vi "Sequence Editor Main.vi"() -> ()   [LabVIEW 2015, in "Configuration Tool.lvlib"]
doc: "This is the main VI for the configuration editor.Copyright 2017 National Instruments Corporation\n\nLicensed under the Apache License, Version 2.0 (the \"License\"); you may not use this file except in compliance with the License. You may obtain a copy of the License at http://www.apache.org/licenses/LICENSE-2.0\nUnless required by applicable law or agreed to in writing, software distributed under the License is distributed on an \"AS IS\" BASIS, WITHOUT WARRANTIES OR CONDITIONS OF ANY KIND, either express or implied. See the License for the specific language governing permissions and limitations under the License."
uses:
  Configuration Tool.lvlib
  Controls/StateCluster.ctl
  <vilib>/NI/Configuration Framework/Repository/NISE_CEF_Repository.lvclass
  <vilib>/NI/Configuration Framework/Node/NodeRef.ctl
  <vilib>/NI/Configuration Framework/Node/NISE_CEF_Node.lvclass
  <vilib>/NI/Configuration Framework/Node/StandardEvents.ctl
  <vilib>/NI/Configuration Framework/Node/UserEventRef.ctl
  <vilib>/NI/Configuration Framework/Controls/EventCluster.ctl
  <vilib>/NI/Configuration Framework/Node/NodeChangeEvent.ctl
  <vilib>/NI/Configuration Framework/Node/CacheState.ctl
  <vilib>/NI/Configuration Framework/Node/RefreshUIEvent.ctl
  <vilib>/NI/Configuration Framework/Node/StopEvent.ctl
  <vilib>/NI/Configuration Framework/glyph manager/glyph manager.ctl
  <vilib>/picture/picture.llb/imagedata.ctl
  Controls/StepClassLibrary.ctl
  Prototype/classes/Step/Config/Step Config.lvclass
  Prototype/classes/Step/UI/Step UI.lvclass
  Controls/AddMessage.ctl
  Controls/MoveMessage.ctl
  <vilib>/Utility/error.llb/DialogType.ctl
  Classes/SequenceNode/SequenceNode.lvclass
  Classes/SequenceRepo/SequenceRepo.lvclass
  <vilib>/Utility/sysdir.llb/System Directory Type.ctl
  Classes/StepNode/StepNode.lvclass
  <vilib>/NI/AMC/Read Termination Message.vi
  <vilib>/NI/AMC/Create Single Message.vi
  <vilib>/NI/AMC/Update Message Routing Info.vi
  <vilib>/NI/AMC/Send Message.vi
  <vilib>/NI/AMC/Globals.vi
  <vilib>/NI/AMC/AMC.lvlib
  <vilib>/NI/Configuration Framework/NISE_CEF_TreeControl.lvlib
  <vilib>/NI/Configuration Framework/glyph manager/glyph manager.lvlib
panel:
  in  "View":string(tree)
  in  "Exit":bool
  # "Configurator"
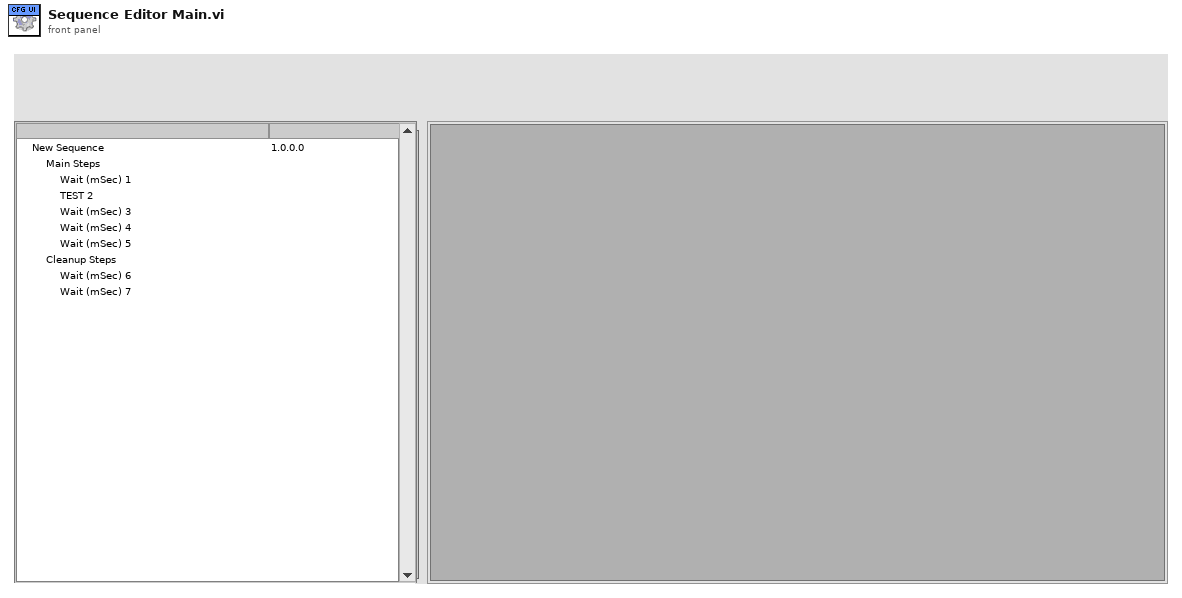
[diagram p1: front panel]
types:
  T1 = typedef "Configuration Tool.lvlib/StateCluster.ctl" = cluster{"repository":refnum<class "NISE_CEF_Repository.lvclass">, "root":T2, "unsaved changes":bool, "current path":path, "standard events":T3, "classes path":path, "glyph manager":T9, "Step Class Library":T11}
  T2 = typedef "NISE_CEF_Node.lvclass/NodeRef.ctl" = refnum<data-value>
  T3 = typedef "NISE_CEF_Node.lvclass/StandardEvents.ctl" = cluster{"user event":T4, "node change":T5, "cache state":T6, "refresh UI":T7, "stop event":T8}
  T4 = typedef "NISE_CEF_Node.lvclass/UserEventRef.ctl" = refnum<user-event>
  T5 = typedef "NISE_CEF_Node.lvclass/NodeChangeEvent.ctl" = refnum<user-event>
  T6 = typedef "NISE_CEF_Node.lvclass/CacheState.ctl" = refnum<user-event>
  T7 = typedef "NISE_CEF_Node.lvclass/RefreshUIEvent.ctl" = refnum<user-event>
  T8 = typedef "NISE_CEF_Node.lvclass/StopEvent.ctl" = refnum<user-event>
  T9 = typedef "glyph manager.lvlib/glyph manager.ctl" = cluster{"search paths":path[], "glyph map":variant, "base glyphs":T10[], "desired overlays":string[]}
  T10 = typedef "imagedata.ctl" = cluster{"image type":i32, "image depth":i32, "image":u8[], "mask":u8[], "colors":u32[], "Rectangle":cluster{"left":i16, "top":i16, "right":i16, "bottom":i16}}
  T11 = typedef "Configuration Tool.lvlib/StepClassLibrary.ctl" = cluster{"Step Types":string[], "Step Config Classes":refnum<class "Step Config.lvclass">[], "Step UI Classes":refnum<class "Step UI.lvclass">[]}
  T12 = typedef "AMC.lvlib/Message Queue.ctl" = refnum<queue>
  T13 = typedef "Configuration Tool.lvlib/AddMessage.ctl" = cluster{"node type":string, "to add to":string}
  T14 = typedef "Configuration Tool.lvlib/MoveMessage.ctl" = cluster{"node ref":T2, "new parent":T2, "Index":i32}
  T15 = typedef "Configuration Tool.lvlib/FilePaths.ctl" = cluster{"glyphs":path, "classes":path}
  T16 = typedef "DialogType.ctl" = u16
  T17 = typedef "System Directory Type.ctl" = i32
  T18 = typedef "NISE_CEF_Node.lvclass/Summary.ctl" = cluster{"ID":string, "parent ID":string, "node type":string, "text":string, "additional text":string, "glyph":string, "depth":i32, "glyph overlay":string}
  T19 = typedef "LVPoint32TypeDef.ctl" = cluster{"Horizontal":i32, "Vertical":i32}
  T20 = cluster{"data name":string, "drag data":variant}[]
  T21 = typedef "NISE_CEF_Node.lvclass/NodeMenuOptions.ctl" = cluster{"removable":bool, "movable":bool, "duplicate":bool}
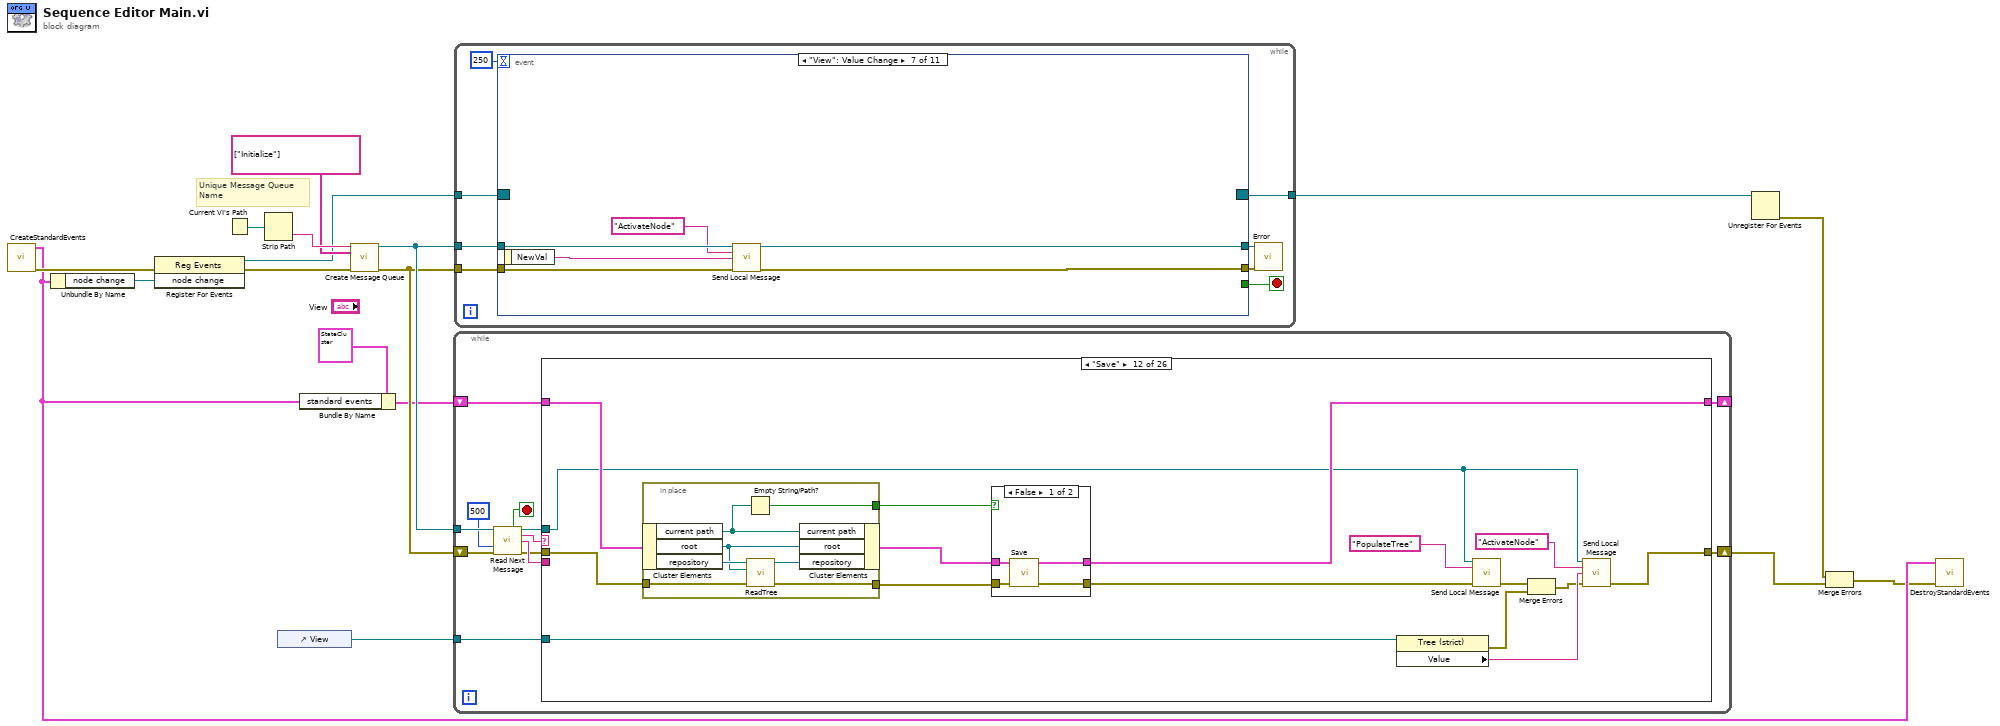
[diagram p0: block diagram]
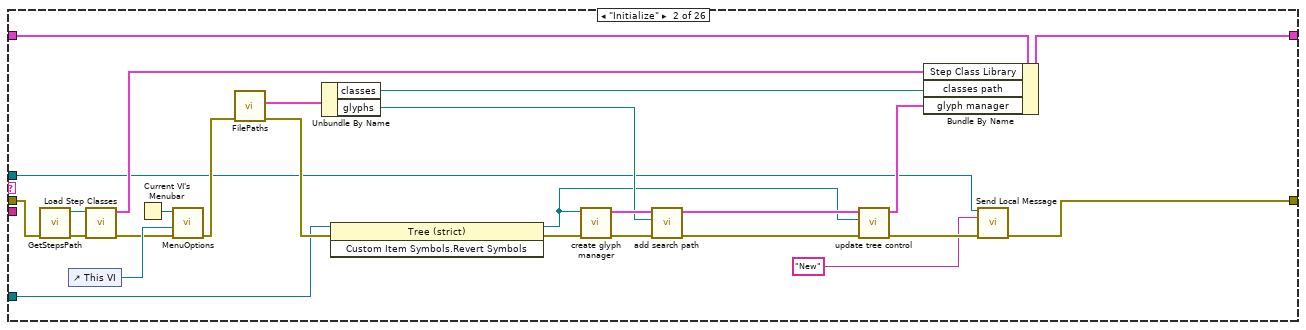
[diagram p3: hidden frame]
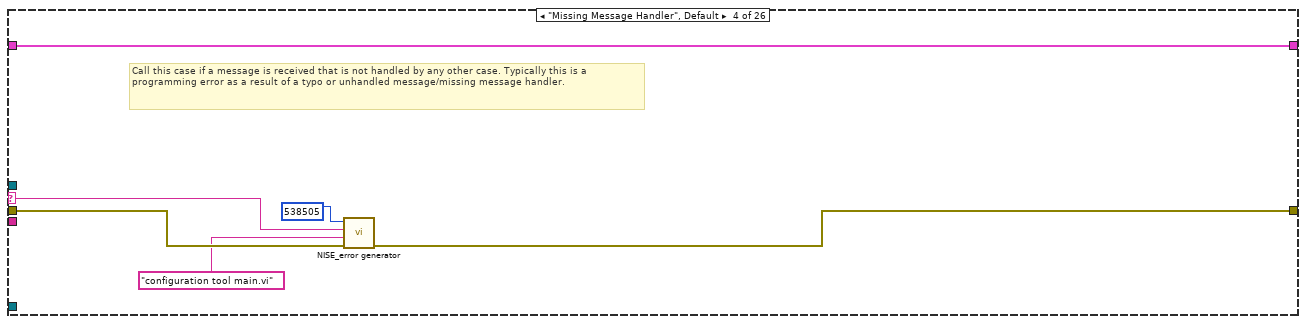
[diagram p5: hidden frame]
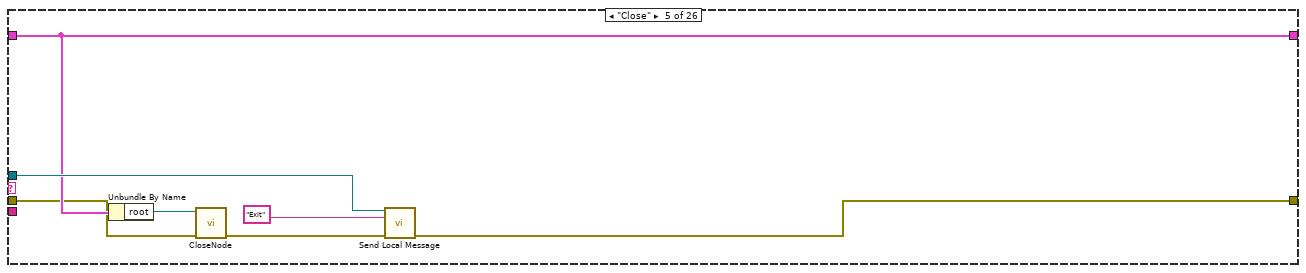
[diagram p6: hidden frame]
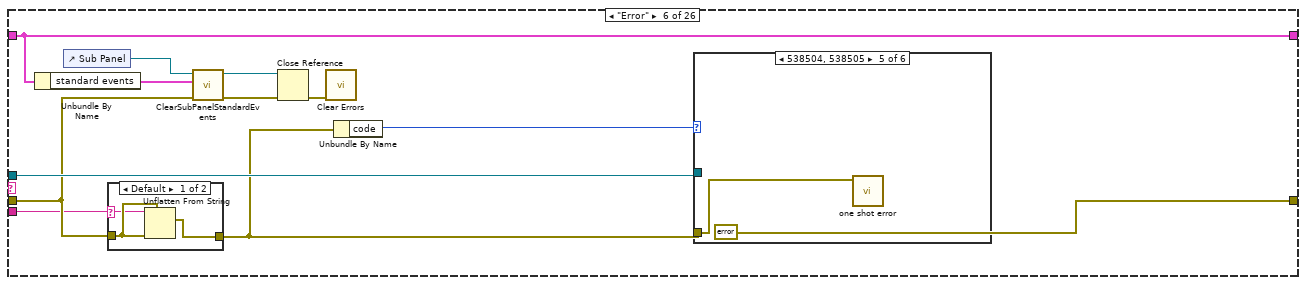
[diagram p7: hidden frame]
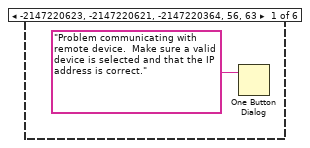
[diagram p9: hidden frame]
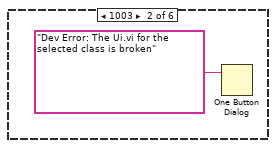
[diagram p10: hidden frame]
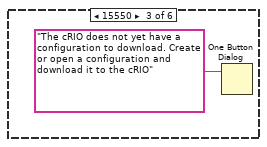
[diagram p11: hidden frame]
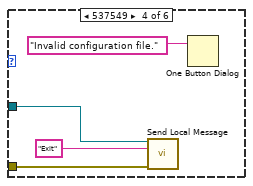
[diagram p12: hidden frame]
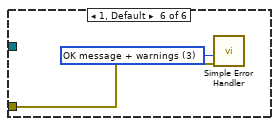
[diagram p13: hidden frame]
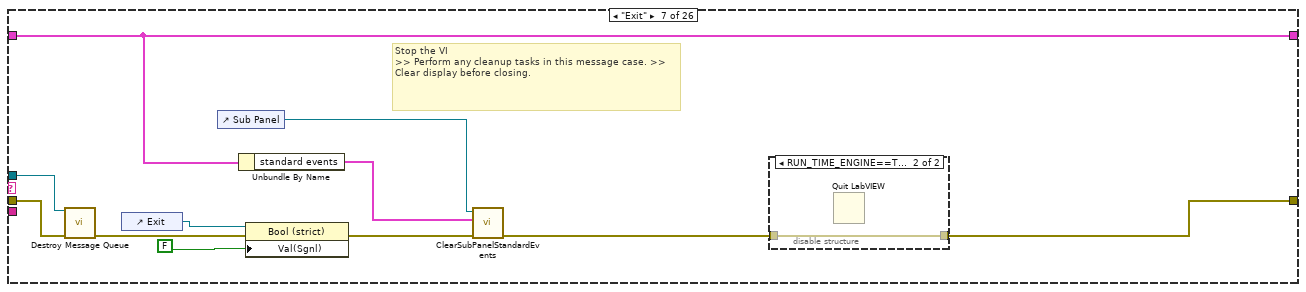
[diagram p14: hidden frame]
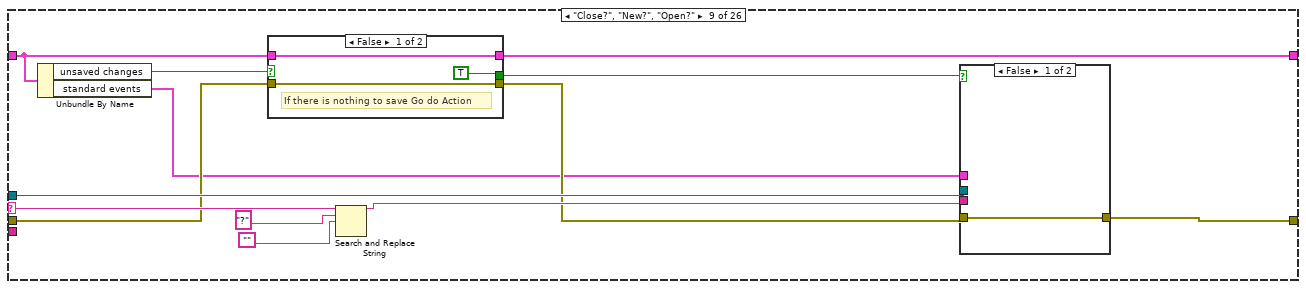
[diagram p17: hidden frame]
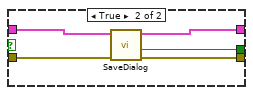
[diagram p18: hidden frame]
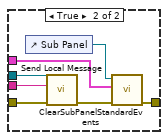
[diagram p19: hidden frame]
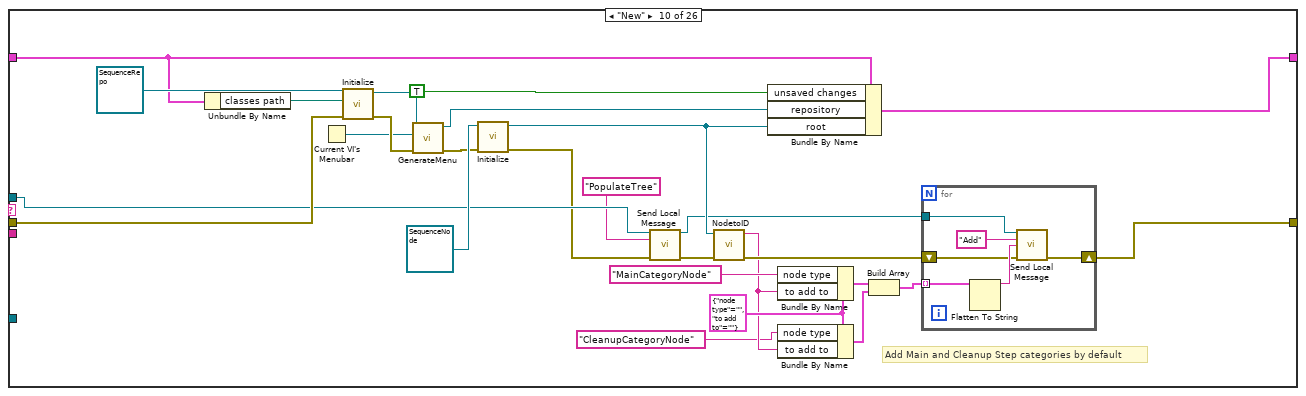
[diagram p20: hidden frame]
diagram:
  # "Unique Message Queue Name"
  n1 = call <vilib>:"CreateStandardEvents.vi"() -> ("error out"=w12:errorcluster, "standard events"=w6:T3)  [unwired: 10 in]
  n2 = Unbundle By Name(w6) -> ("node change"=w11:T5)
  n3 = register-events(error in=w12, w11) -> (reference out=w5:refnum<event-registration>, error out=w10:errorcluster)  [unwired: 1 in]
  n4 = Current VI's Path() -> (path=w16:path)
  n5 = Strip Path(path=w16) -> (name=w17:string)  [unwired: 1 out]
  n6 = control-ref of="View"() -> (w4:refnum<vi>)
  n7 = Bundle By Name(cluster=T1 {"repository"=refnum, "root"=refnum, "unsaved changes"=FALSE, "current path"=path "", "standard events"={"user event"=refnum, "node change"=refnum, "cache state"=refnum, "refresh UI"=refnum, "stop event"=refnum}, "classes path"=path "", "glyph manager"={"search paths"=[], "glyph map"=variant, "base glyphs"=[], "desired overlays"=[]}, "Step Class Library"={"Step Types"=[], "Step Config Classes"=[], "Step UI Classes"=[]}}, "standard events"=w6) -> (w8:T1)
  n8 = call <vilib>:"Create Message Queue.vi"("message queue name"=w17, "initial message names"=string[] ["Initialize"], "error in"=w10) -> ("message queue out"=w14:T12, "error out"=w13:errorcluster)  [unwired: 11 in]
  n9 = while "Message Processor" {
    shift-right: [w25] -> w7
    shift-left: w13 -> [w24]
    tunnel: w14 -> [w23]
    shift-right: [w21] -> _
    shift-left: w8 -> [w20]
    tunnel: w4 -> [w18]
    stop <- w29 stop-if-true
    n10 = call <vilib>:"Read Next Message.vi"("message queue in"=w23, "timeout (1 ms)"=500, "error in"=w24) -> ("exit process?"=w29:bool, "message queue out"=w19:T12, "message name"=w28:string, "message value"=w27:string, "error out"=w26:errorcluster)  [unwired: 5 in, 3 out]
    n11 = case shown="\"Save\"" w28 {
      selector: w28 -> [_ _ _ w61 _ _ _ _ w122 _ _ _ _ _ _ _ _ _ w423 _ _ _ _ _ _ _]
      tunnel: w27 -> [_ _ _ _ _ w74 _ _ _ _ _ _ _ w262 _ w311 w370 w401 w421 w473 w497 _ _ w537 w558 w565]
      tunnel: w26 -> [w31 w35 w59 w64 w67 w77 w109 w113 w115 w163 w182 w229 w254 w269 w282 w303 w365 w400 w426 w475 w496 w518 w527 w536 w556 w566]
      tunnel: [w31 w34 w59 w62 w71 errorcluster {"status"=FALSE, "code"=0, "source"=""} ("error out") w101 w113 w126 w156 w178 w225 w256 w266 w282 w305 w336 w404 w429 w477 w493 w512 w523 w533 w551 w564] -> w25
      tunnel: [w30 w53 w58 w65 w69 w81 w100 w112 w117 w169 w183 w235 w255 w263 w281 w298 w360 w397 w430 w476 w498 w509 w526 w531 w559 w561] -> w21
      tunnel: w20 -> [w30 w54 w58 w65 w69 w81 w100 w112 w118 w165 w184 w231 w253 w264 w281 w301 w363 w398 w430 w468 w498 w521 w526 w531 w559 w567]
      tunnel: w19 -> [_ w33 _ _ w70 w84 w108 _ w125 w154 w180 w223 _ w265 _ _ w335 _ w424 _ _ _ _ w532 w550 w563]
      tunnel: w18 -> [_ w40 _ _ _ _ _ _ _ _ _ w226 _ _ _ w299 w361 w393 w418 w470 w491 w510 _ _ _ _]
      frame "------------Generic Operations------------" {
        # "Dummy case to add a seperation in the Case Structure menu"
      }
      frame "Initialize" {
        n12 = call "GetStepsPath.vi"("error in (no error)"=w35) -> ("error out"=w36:errorcluster, "Steps Folder Path"=w37:path)  [unwired: 9 in]
        n13 = control-ref of="This VI"() -> (w57:refnum<vi>)
        n14 = call "Load Step Classes.vi"("error in (no error)"=w36, "Step Classes Folder Path"=w37) -> ("error out"=w39:errorcluster, "Step Class Library"=w38:T11)  [unwired: 8 in]
        n15 = Current VI's Menubar() -> (w56:refnum<k9>)
        n16 = call "MenuOptions.vi"("error in"=w39, "VI ref"=w57, "menu ref in"=w56) -> ("error out"=w52:errorcluster)  [unwired: 7 in, 1 out]
        n17 = call "FilePaths.vi"("error in"=w52) -> ("error out"=w43:errorcluster, "paths"=w55:T15)  [unwired: 9 in]
        n18 = Unbundle By Name(w55) -> ("classes"=w51:path, "glyphs"=w45:path)
        n19 = invoke class="Tree (strict)" method="Custom Item Symbols.Revert Symbols"(reference=w40, error in=w43) -> (reference out=w41:refnum<vi>, error out=w42:errorcluster)  [unwired: 1 in, 1 out]
        n20 = call <vilib>:"create glyph manager.vi"("error in"=w42, "tree ref (for default symbols)"=w41) -> ("error out"=w50:errorcluster, "glyph manager"=w49:T9)  [unwired: 8 in]
        n21 = call <vilib>:"add search path.vi"("error in"=w50, "search path"=w45, "glyph manager in"=w49) -> ("error out"=w48:errorcluster, "glyph manager out"=w47:T9)  [unwired: 7 in]
        n22 = call <vilib>:"update tree control.vi"("error in"=w48, "tree reference"=w41, "glyph manager in"=w47) -> ("error out"=w46:errorcluster, "glyph manager out"=w44:T9)  [unwired: 7 in]
        n23 = Bundle By Name(cluster=w54, "Step Class Library"=w38, "classes path"=w51, "glyph manager"=w44) -> (w53:T1)
        n24 = call <vilib>:"Send Local Message.vi"("message queue in"=w33, "message name"="New", "error in"=w46) -> ("error out"=w34:errorcluster)  [unwired: 10 in, 2 out]
      }
      frame "", "Idle" {
      }
      frame "Missing Message Handler", Default {
        # "Call this case if a message is received that is not handled by any other case. Typically this is a programming error as a result of a typo or unhandled message/missing message handler."
        n25 = call <vilib>:"NISE_error generator.vi"("error in"=w64, "source"="configuration tool main.vi", "append error message"=w61, "error code (0)"=538505) -> ("error out"=w62:errorcluster)  [unwired: 5 in]
      }
      frame "Close" {
        n26 = Unbundle By Name(w69) -> ("root"=w68:T2)
        n27 = call <vilib>:"CloseNode.vi"("error in"=w67, "node ref"=w68) -> ("error out"=w66:errorcluster)  [unwired: 9 in]
        n28 = call <vilib>:"Send Local Message.vi"("message queue in"=w70, "message name"="Exit", "error in"=w66) -> ("error out"=w71:errorcluster)  [unwired: 10 in, 2 out]
      }
      frame "Error" {
        n29 = Unbundle By Name(w81) -> ("standard events"=w73:T3)
        n30 = control-ref of="Sub Panel"() -> (w80:refnum<vi>)
        n31 = case shown="Default" w74 {
          selector: w74 -> [w86 _]
          tunnel: w77 -> [w87 w88]
          tunnel: [w85 w88] -> w76
          frame Default {
            n32 = Unflatten From String(type=w87, binary string=w86, error in (no error)=w87) -> (value=w85:errorcluster)  [unwired: 2 in, 2 out]
          }
          frame "" {
          }
        }
        n33 = call <vilib>:"ClearSubPanelStandardEvents.vi"("error in"=w77, "standard events"=w73, "sub panel ref in"=w80) -> ("error out"=w79:errorcluster, "sub panel ref out"=w78:refnum<vi>)  [unwired: 7 in]
        n34 = Close Reference(reference=w78, error in (no error)=w79) -> (error out=w75:errorcluster)
        n35 = call <vilib>:"Clear Errors.vi"("error in (no error)"=w75) -> ()  [unwired: 5 in, 2 out]
        n36 = Unbundle By Name(w76) -> ("code"=w82:i32)
        n37 = case shown="538504, 538505" w82 {
          tunnel: w84 -> [_ _ _ w94 _ _]
          tunnel: w76 -> [_ _ _ w93 w96 w98]
          frame -2147220623, -2147220621, -2147220364, 56, 63 {
            n38 = One Button Dialog(message="Problem communicating with remote device.  Make sure a valid device is selected and that the IP address is correct.") -> ()  [unwired: 1 in, 1 out]
          }
          frame 1003 {
            n39 = One Button Dialog(message="Dev Error: The Ui.vi for the selected class is broken") -> ()  [unwired: 1 in, 1 out]
          }
          frame 15550 {
            n40 = One Button Dialog(message="The cRIO does not yet have a configuration to download. Create or open a configuration and download it to the cRIO") -> ()  [unwired: 1 in, 1 out]
          }
          frame 537549 {
            n41 = call <vilib>:"Send Local Message.vi"("message queue in"=w94, "message name"="Exit", "error in"=w93) -> ()  [unwired: 10 in, 3 out]
            n42 = One Button Dialog(message="Invalid configuration file.") -> ()  [unwired: 1 in, 1 out]
          }
          frame 538504, 538505 {
            n43 = call <vilib>:"one shot error.vi"("error in"=w96) -> ()  [unwired: 11 in]
          }
          frame 1, Default {
            w97 = T16 3 items=["no dialog", "OK message", "continue or stop message", "OK message + warnings", "continue/stop + warnings"] ("type of dialog (OK msg:1)")
            n44 = call <vilib>:"Simple Error Handler.vi"("type of dialog (OK msg:1)"=w97, "error in (no error)"=w98) -> ()  [unwired: 8 out]
          }
        }
      }
      frame "Exit" {
        # "Stop the VI                                                                             >> Perform any cleanup tasks in this message case. >> Clear display before closing."
        n45 = call <vilib>:"Destroy Message Queue.vi"("message queue in"=w108, "error in"=w109) -> ("error out"=w105:errorcluster)  [unwired: 11 in, 2 out]
        n46 = control-ref of="Exit"() -> (w107:refnum<vi>)
        n47 = control-ref of="Sub Panel"() -> (w104:refnum<vi>)
        n48 = Unbundle By Name(w100) -> ("standard events"=w99:T3)
        n49 = property class="Bool (strict)"(reference=w107, error in=w105, "Val(Sgnl)"=FALSE ("Exit")) -> (error out=w103:errorcluster)  [unwired: 1 out]
        n50 = call <vilib>:"ClearSubPanelStandardEvents.vi"("error in"=w103, "standard events"=w99, "sub panel ref in"=w104) -> ("error out"=w102:errorcluster)  [unwired: 7 in, 1 out]
        n51 = disable-structure shown="RUN_TIME_ENGINE==True" {
          disable-tunnel: [w110 w111] -> w101
          disable-tunnel: w102 -> [w110 w111]
          frame condition #0 (active) {
          }
          frame condition #1 {
            n52 = Quit LabVIEW() -> ()  [unwired: 1 in]
          }
        }
      }
      frame "------------Menu Operations--------------" {
        # "Dummy case to add a seperation in the Case Structure menu"
      }
      frame "Close?", "New?", "Open?" {
        n53 = Unbundle By Name(w118) -> ("unsaved changes"=w120:bool, "standard events"=w114:T3)
        n54 = case shown="False" w120 {
          tunnel: [TRUE ("SaveFlag") w134] -> w119
          tunnel: w118 -> [w128 w133]
          tunnel: [w128 w132] -> w117
          tunnel: w115 -> [w127 w131]
          tunnel: [w127 w130] -> w116
          frame False {
            # "If there is nothing to save Go do Action"
          }
          frame True {
            n55 = call "SaveDialog.vi"("error in"=w131, "state in"=w133) -> ("error out"=w130:errorcluster, "new"=w134:bool, "state out"=w132:T1)  [unwired: 7 in]
          }
        }
        n56 = Search and Replace String(input string=w122, search string="?", replace string="") -> (result string=w121:string)  [unwired: 5 in, 3 out]
        n57 = case shown="False" w119 {
          tunnel: w116 -> [w135 w142]
          tunnel: [w135 w138] -> w126
          tunnel: w125 -> [_ w141]
          tunnel: w121 -> [_ w140]
          tunnel: w114 -> [_ w136]
          frame False {
          }
          frame True {
            n58 = control-ref of="Sub Panel"() -> (w137:refnum<vi>)
            n59 = call <vilib>:"Send Local Message.vi"("message queue in"=w141, "message name"=w140, "error in"=w142) -> ("error out"=w139:errorcluster)  [unwired: 10 in, 2 out]
            n60 = call <vilib>:"ClearSubPanelStandardEvents.vi"("error in"=w139, "standard events"=w136, "sub panel ref in"=w137) -> ("error out"=w138:errorcluster)  [unwired: 7 in, 1 out]
          }
        }
      }
      frame "New" {
        w146 = T13 {"node type"="", "to add to"=""} ("input cluster")
        # "Add Main and Cleanup Step categories by default"
        n61 = Unbundle By Name(w165) -> ("classes path"=w164:path)
        n62 = Current VI's Menubar() -> (w158:refnum<k9>)
        n63 = call-dynamic "Initialize.vi"("error in"=w163, "path"=w164, "repository in"=refnum<class "SequenceRepo.lvclass"> refnum ("cRIORepo.lvclass")) -> ("error out"=w162:errorcluster, "repository out"=w160:refnum<class "SequenceRepo.lvclass">)  [unwired: 7 in]
        n64 = call-dynamic "GenerateMenu.vi"("error in"=w162, "menu ref in"=w158, "NISE_CEF_Repository in"=w160) -> ("error out"=w161:errorcluster, "NISE_CEF_Repository out"=w159:refnum<class "SequenceRepo.lvclass">)  [unwired: 6 in, 1 out]
        n65 = call-dynamic "Initialize.vi"("error in"=w161, "SequenceNode in"=refnum<class "SequenceNode.lvclass"> refnum ("cRIO.lvclass")) -> ("error out"=w151:errorcluster, "data value reference"=w157:T2)  [unwired: 7 in, 1 out]
        n66 = call <vilib>:"Send Local Message.vi"("message queue in"=w154, "message name"="PopulateTree", "error in"=w151) -> ("message queue out"=w153:T12, "error out"=w150:errorcluster)  [unwired: 10 in, 1 out]
        n67 = call <vilib>:"NodetoID.vi"("error in"=w150, "node ref"=w157) -> ("error out"=w149:errorcluster, "ID"=w144:string)  [unwired: 8 in]
        n68 = Bundle By Name(cluster=w165, "unsaved changes"=TRUE ("SaveFlag"), "repository"=w159, "root"=w157) -> (w169:T1)
        n69 = Bundle By Name(cluster=w146, "node type"="MainCategoryNode", "to add to"=w144) -> (w147:T13)
        n70 = Bundle By Name(cluster=w146, "node type"="CleanupCategoryNode", "to add to"=w144) -> (w145:T13)
        n71 = Build Array(w147, w145) -> (w148:T13[])
        n72 = for {
          tunnel: w148 -> [w173] mode=indexing
          tunnel: w153 -> [w171]
          shift-right: [w175] -> w156
          shift-left: w149 -> [w170]
          n73 = Flatten To String(anything=w173) -> (data string=w172:string)  [unwired: 3 in, 2 out]
          n74 = call <vilib>:"Send Local Message.vi"("message queue in"=w171, "message name"="Add", "message value"=w172, "error in"=w170) -> ("error out"=w175:errorcluster)  [unwired: 9 in, 2 out]
        }
      }
      frame "Open" {
        w177 = T17 0 items=["User Home"=0, "User Desktop"=1, "User Documents"=2, "User Application Data"=3, "User Preferences"=4, "User Temporary"=5, "Public Documents"=6, "Public Application Data"=7, "Public Preferences"=8, "Public Cache"=13, "System Core Libraries"=9, "System Installed Libraries"=10, "Application Files"=11, "Boot Volume Root"=12] ("system directory type")
        n75 = call <vilib>:"Get System Directory.vi"("system directory type"=w177) -> ("system directory"=w176:path)  [unwired: 10 in]
        n76 = in-place {
          in-place-border: w182 -> [w190]
          in-place-border: [w189] -> w179
          in-place-border: w176 -> [w185]
          n77 = in-place-cluster #1(w184) -> ("current path"=w187:path, "repository"=w198:refnum<class "NISE_CEF_Repository.lvclass">, "root"=w194:T2)  [unwired: 1 out]
          n78 = call "FileDialog.vi"("error in"=w190, "start path"=w185) -> ("error out"=w191:errorcluster, "cancelled"=w192:bool, "selected path"=w188:path)  [unwired: 7 in]
          n79 = Compound Arithmetic op=OR(invert w192) -> (w193:bool)
          n80 = case shown="True" w193 {
            tunnel: w198 -> [w199 w211]
            tunnel: [w199 w209] -> w196
            tunnel: [w200 w207] -> w189
            tunnel: [w201 w206] -> w195
            tunnel: w188 -> [_ w204]
            tunnel: w191 -> [w200 w203]
            tunnel: w194 -> [w201 w202]
            frame False {
            }
            frame True {
              n81 = call-dynamic "Open.vi"("error in"=w203, "file path"=w204, "repository in"=w211) -> ("error out"=w208:errorcluster, "invalid?"=w205:bool, "repository out"=w210:refnum<class "NISE_CEF_Repository.lvclass">)  [unwired: 6 in]
              n82 = case shown="False" w205 {
                tunnel: w210 -> [w216 w219]
                tunnel: [w215 w219] -> w209
                tunnel: w208 -> [w214 w218]
                tunnel: [w213 w218] -> w207
                tunnel: [w212 w217] -> w206
                tunnel: w202 -> [_ w217]
                frame False {
                  n83 = call-dynamic "WriteTree.vi"("error in"=w214, "repository in"=w216) -> ("error out"=w213:errorcluster, "root"=w212:T2, "repository out"=w215:refnum<class "NISE_CEF_Repository.lvclass">)  [unwired: 7 in]
                }
                frame True {
                }
              }
            }
          }
          n84 = Select(t=w187, s=w189, f=w188) -> (s? t:f=w186:path)
          n85 = in-place-cluster #1("current path"=w186, "unsaved changes"=FALSE ("SaveFlag"), "repository"=w196, "root"=w195) -> (w183:T1)
        }
        n86 = call <vilib>:"Send Local Message.vi"("message queue in"=w180, "message name"="PopulateTree", "error in"=w179) -> ("error out"=w178:errorcluster)  [unwired: 10 in, 2 out]
      }
      frame "Save" {
        n87 = in-place {
          in-place-border: w229 -> [w239]
          in-place-border: [w238] -> w228
          in-place-border: [w236] -> w227
          n88 = in-place-cluster #2(w231) -> ("current path"=w237:path, "root"=w240:T2, "repository"=w242:refnum<class "NISE_CEF_Repository.lvclass">)
          n89 = Empty String/Path?(string/path=w237) -> (empty?=w236:bool)
          n90 = call-dynamic "ReadTree.vi"("error in"=w239, "root"=w240, "repository in"=w242) -> ("error out"=w238:errorcluster, "repository out"=w241:refnum<class "NISE_CEF_Repository.lvclass">)  [unwired: 7 in]
          n91 = in-place-cluster #2("current path"=w237, "root"=w240, "repository"=w241) -> (w230:T1)
        }
        n92 = case shown="False" w227 {
          tunnel: w230 -> [w246 w248]
          tunnel: [w245 w247] -> w235
          tunnel: [w244 w249] -> w233
          tunnel: w228 -> [w243 w250]
          frame False {
            n93 = call "Save.vi"("error in"=w243, "state in"=w246) -> ("error out"=w244:errorcluster, "state out"=w245:T1)  [unwired: 8 in]
          }
          frame True {
            # "Empty path use Dialog"
            n94 = call "SaveAs.vi"("error in"=w250, "state in"=w248) -> ("error out"=w249:errorcluster, "state out"=w247:T1)  [unwired: 7 in, 1 out]
          }
        }
        n95 = property class="Tree (strict)"(reference=w226) -> (error out=w220:errorcluster, "Value"=w222:string)  [unwired: 1 in, 1 out]
        n96 = call <vilib>:"Send Local Message.vi"("message queue in"=w223, "message name"="PopulateTree", "error in"=w233) -> ("error out"=w232:errorcluster)  [unwired: 10 in, 2 out]
        n97 = Merge Errors(w232, w220) -> (w221:errorcluster)
        n98 = call <vilib>:"Send Local Message.vi"("message queue in"=w223, "message name"="ActivateNode", "message value"=w222, "error in"=w221) -> ("error out"=w225:errorcluster)  [unwired: 9 in, 2 out]
      }
      frame "SaveAs" {
        n99 = in-place {
          in-place-border: w254 -> [w258]
          in-place-border: [w257] -> w252
          n100 = in-place-cluster #3(w253) -> ("root"=w259:T2, "repository"=w261:refnum<class "NISE_CEF_Repository.lvclass">)
          n101 = call-dynamic "ReadTree.vi"("error in"=w258, "root"=w259, "repository in"=w261) -> ("error out"=w257:errorcluster, "repository out"=w260:refnum<class "NISE_CEF_Repository.lvclass">)  [unwired: 7 in]
          n102 = in-place-cluster #3("root"=w259, "repository"=w260) -> (w251:T1)
        }
        n103 = call "SaveAs.vi"("error in"=w252, "state in"=w251) -> ("error out"=w256:errorcluster, "state out"=w255:T1)  [unwired: 7 in, 1 out]
      }
      frame "Custom View" {
        n104 = in-place {
          in-place-border: w269 -> [w280]
          in-place-border: [w279] -> w267
          in-place-border: w262 -> [w270]
          n105 = in-place-cluster #4(w264) -> ("repository"=w274:refnum<class "NISE_CEF_Repository.lvclass">, "root"=w273:T2)
          n106 = call-dynamic "ReadTree.vi"("error in"=w280, "root"=w273, "repository in"=w274) -> ("error out"=w277:errorcluster, "repository out"=w276:refnum<class "NISE_CEF_Repository.lvclass">)  [unwired: 7 in]
          n107 = call-dynamic "CustomView.vi"("error in"=w277, "view name"=w270, "repository in"=w276) -> ("error out"=w278:errorcluster, "repository out"=w275:refnum<class "NISE_CEF_Repository.lvclass">)  [unwired: 7 in]
          n108 = call-dynamic "WriteTree.vi"("error in"=w278, "repository in"=w275) -> ("error out"=w279:errorcluster, "root"=w271:T2, "repository out"=w272:refnum<class "NISE_CEF_Repository.lvclass">)  [unwired: 7 in]
          n109 = in-place-cluster #4("repository"=w272, "root"=w271) -> (w263:T1)
        }
        n110 = call <vilib>:"Send Local Message.vi"("message queue in"=w265, "message name"="PopulateTree", "error in"=w267) -> ("error out"=w266:errorcluster)  [unwired: 10 in, 2 out]
      }
      frame "-------TreeControl Operations-----------" {
        # "Dummy case to add a seperation in the Case Structure menu"
      }
      frame "Add" {
        # "Load specific step class"
        n111 = Unflatten From String(type=T13 {"node type"="", "to add to"=""} ("input cluster"), binary string=w311) -> (value=w309:T13)  [unwired: 3 in, 2 out]
        n112 = Unbundle By Name(w309) -> ("to add to"=w307:string, "node type"=w290:string)
        n113 = Match Pattern(string=w290, regular expression=":") -> (before substring=w289:string, after substring=w288:string)  [unwired: 1 in, 2 out]
        n114 = in-place {
          in-place-border: w303 -> [w328]
          in-place-border: [w327] -> w302
          in-place-border: [w326] -> w300
          in-place-border: w289 -> [w325]
          n115 = in-place-cluster #5(w301) -> ("repository"=w330:refnum<class "NISE_CEF_Repository.lvclass">)
          n116 = call-dynamic "GetClassPath.vi"("error in"=w328, "class name"=w325, "Repository in"=w330) -> ("error out"=w327:errorcluster, "class path"=w326:path, "Repository out"=w329:refnum<class "NISE_CEF_Repository.lvclass">)  [unwired: 6 in]
          n117 = in-place-cluster #5("repository"=w329) -> (w284:T1)
        }
        n118 = Unbundle By Name(w284) -> ("glyph manager"=w296:T9)
        n119 = Unbundle By Name(w284) -> ("Step Class Library"=w283:T11)
        n120 = call <vilib>:"Get LV Class Default Value.vi"("error in (no error)"=w302, "class path"=w300) -> ("error out"=w312:errorcluster, "object"=w313:refnum<class>)  [unwired: 8 in]
        n121 = To More Specific Class(target class=refnum<class "NISE_CEF_Node.lvclass"> refnum ("Node.lvclass"), reference=w313, error in=w312) -> (specific class reference=w285:refnum<class "NISE_CEF_Node.lvclass">, error out=w297:errorcluster)
        n122 = case shown="Default" w288 {
          selector: w288 -> [_ w318]
          tunnel: w297 -> [w315 w324]
          tunnel: [w315 w323] -> w287
          tunnel: [w314 w322] -> w286
          tunnel: w285 -> [w314 w320]
          tunnel: w283 -> [_ w316]
          frame "" {
          }
          frame Default {
            n123 = To More Specific Class(target class=refnum<class "StepNode.lvclass"> refnum ("StepNode.lvclass"), reference=w320, error in=w324) -> (specific class reference=w319:refnum<class "StepNode.lvclass">, error out=w321:errorcluster)
            n124 = call-dynamic "LoadStepType.vi"("error in (no error)"=w321, "Step Class Library"=w316, "Step Type"=w318, "StepNode in"=w319) -> ("error out"=w323:errorcluster, "StepNode out"=w322:refnum<class "StepNode.lvclass">)  [unwired: 6 in]
          }
        }
        n125 = call-dynamic "AddGlyphtoGManager.vi"("error in"=w287, "glyph manager"=w296, "NISE_CEF_Node in"=w286) -> ("error out"=w294:errorcluster, "glyph manager out"=w295:T9, "NISE_CEF_Node out"=w293:refnum<class "NISE_CEF_Node.lvclass">)  [unwired: 6 in]
        n126 = call <vilib>:"AddNode.vi"("error in"=w294, "node in"=w293, "parent node ID"=w307) -> ("error out"=w306:errorcluster, "summary"=w304:T18[])  [unwired: 7 in]
        n127 = call <vilib>:"PopulateTreeSumaryWithGlyphManager.vi"("error in"=w306, "glyph manager"=w295, "summary"=w304, "tree ref in"=w299) -> ("error out"=w305:errorcluster, "glyph manager out"=w292:T9)  [unwired: 6 in]
        n128 = Bundle By Name(cluster=w284, "glyph manager"=w292) -> (w298:T1)
      }
      frame "AddPeer" {
        w332 = ":" ("regular expression")
        # "Load specific step class"
        # "Load \"StepNode\""
        # "Source Node"
        # "Parse \"Before\"/\"After\""
        n129 = Unflatten From String(type=T13 {"node type"="", "to add to"=""} ("input cluster"), binary string=w370) -> (value=w368:T13)  [unwired: 3 in, 2 out]
        n130 = Unbundle By Name(w368) -> ("to add to"=w341:string, "node type"=w348:string)
        n131 = Match Pattern(string=w348, regular expression=w332) -> (before substring=w337:string, after substring=w347:string)  [unwired: 1 in, 2 out]
        n132 = Match Pattern(string=w347, regular expression=w332) -> (before substring=w354:string, after substring=w333:string)  [unwired: 1 in, 2 out]
        n133 = in-place {
          in-place-border: w365 -> [w390]
          in-place-border: [w389] -> w364
          in-place-border: [w388] -> w362
          in-place-border: w354 -> [w387]
          n134 = in-place-cluster #6(w363) -> ("repository"=w392:refnum<class "NISE_CEF_Repository.lvclass">)
          n135 = call-dynamic "GetClassPath.vi"("error in"=w390, "class name"=w387, "Repository in"=w392) -> ("error out"=w389:errorcluster, "class path"=w388:path, "Repository out"=w391:refnum<class "NISE_CEF_Repository.lvclass">)  [unwired: 6 in]
          n136 = in-place-cluster #6("repository"=w391) -> (w350:T1)
        }
        n137 = Match Pattern(string=w333, regular expression=w332) -> (before substring=w331:string)  [unwired: 1 in, 3 out]
        n138 = Unbundle By Name(w350) -> ("glyph manager"=w358:T9)
        n139 = Unbundle By Name(w350) -> ("Step Class Library"=w349:T11)
        n140 = call <vilib>:"Get LV Class Default Value.vi"("error in (no error)"=w364, "class path"=w362) -> ("error out"=w371:errorcluster, "object"=w372:refnum<class>)  [unwired: 8 in]
        n141 = To More Specific Class(target class=refnum<class "NISE_CEF_Node.lvclass"> refnum ("Node.lvclass"), reference=w372, error in=w371) -> (specific class reference=w351:refnum<class "NISE_CEF_Node.lvclass">, error out=w359:errorcluster)
        n142 = case shown="Default" w331 {
          selector: w331 -> [_ w380]
          tunnel: w359 -> [w377 w386]
          tunnel: [w377 w385] -> w353
          tunnel: [w376 w384] -> w352
          tunnel: w351 -> [w376 w382]
          tunnel: w349 -> [_ w378]
          frame "" {
          }
          frame Default {
            n143 = To More Specific Class(target class=refnum<class "StepNode.lvclass"> refnum ("StepNode.lvclass"), reference=w382, error in=w386) -> (specific class reference=w381:refnum<class "StepNode.lvclass">, error out=w383:errorcluster)
            n144 = call-dynamic "LoadStepType.vi"("error in (no error)"=w383, "Step Class Library"=w378, "Step Type"=w380, "StepNode in"=w381) -> ("error out"=w385:errorcluster, "StepNode out"=w384:refnum<class "StepNode.lvclass">)  [unwired: 6 in]
          }
        }
        n145 = call-dynamic "AddGlyphtoGManager.vi"("error in"=w353, "glyph manager"=w358, "NISE_CEF_Node in"=w352) -> ("error out"=w356:errorcluster, "glyph manager out"=w357:T9, "NISE_CEF_Node out"=w340:refnum<class "NISE_CEF_Node.lvclass">)  [unwired: 6 in]
        n146 = call "Get TreeIndex from ID.vi"("error in (no error)"=w356, "Node ID"=w341) -> ("error out"=w342:errorcluster, "TreeIndex"=w339:i32)  [unwired: 8 in]
        n147 = case shown="\"Before\"" w337 {
          tunnel: w339 -> [w373 w375]
          tunnel: [w373 w374] -> w338
          frame "Before" {
          }
          frame "After", Default {
            n148 = Increment(x=w375) -> (x+1=w374:i32)
          }
        }
        n149 = call "Get Parent Node ID from ID.vi"("error in (no error)"=w342, "Node ID"=w341) -> ("error out"=w346:errorcluster, "Parent ID"=w345:string)  [unwired: 8 in]
        n150 = call "AddPeerNodeAtIndex.vi"("error in"=w346, "TreeIndex"=w338, "parent node ID"=w345, "node in"=w340) -> ("error out"=w343:errorcluster, "summary"=w344:T18[])  [unwired: 6 in]
        n151 = call <vilib>:"PopulateTreeSumaryWithGlyphManager.vi"("error in"=w343, "glyph manager"=w357, "summary"=w344, "tree ref in"=w361) -> ("error out"=w366:errorcluster, "glyph manager out"=w355:T9)  [unwired: 6 in]
        n152 = Bundle By Name(cluster=w350, "glyph manager"=w355) -> (w360:T1)
        n153 = call <vilib>:"Send Local Message.vi"("message queue in"=w335, "message name"="PopulateTree", "error in"=w366) -> ("error out"=w336:errorcluster)  [unwired: 10 in, 2 out]
      }
      frame "Duplicate" {
        n154 = call <vilib>:"IDtoNode.vi"("error in"=w400, "ID"=w401) -> ("error out"=w402:errorcluster, "invalid Id"=w399:bool, "node ref"=w403:T2)  [unwired: 7 in]
        n155 = Unbundle By Name(w398) -> ("glyph manager"=w395:T9)
        n156 = case shown="False" w399 {
          tunnel: [w415 w417] -> w404
          tunnel: w403 -> [w414 _]
          tunnel: w402 -> [w411 w417]
          tunnel: w395 -> [w407 w416]
          tunnel: [w406 w416] -> w394
          tunnel: w393 -> [w405 _]
          frame False {
            n157 = call <vilib>:"DuplicateNode.vi"("same parent?"=TRUE ("s"), "error in"=w411, "node ref in"=w414) -> ("error out"=w412:errorcluster, "new node ref"=w413:T2)  [unwired: 7 in]
            n158 = call <vilib>:"Summary.vi"("error in"=w412, "node self ref"=w413) -> ("error out"=w409:errorcluster, "summary"=w408:T18[])  [unwired: 8 in]
            n159 = call <vilib>:"PopulateTreeSumaryWithGlyphManager.vi"("error in"=w409, "glyph manager"=w407, "summary"=w408, "tree ref in"=w405) -> ("error out"=w415:errorcluster, "glyph manager out"=w406:T9)  [unwired: 6 in]
          }
          frame True {
          }
        }
        n160 = Bundle By Name(cluster=w398, "unsaved changes"=TRUE, "glyph manager"=w394) -> (w397:T1)
      }
      frame "CustomMenuAction" {
        n161 = Match Pattern(string=w421, regular expression=":") -> (before substring=w420:string, after substring=w419:string)  [unwired: 1 in, 2 out]
        n162 = call <vilib>:"IDtoNode.vi"("error in"=w426, "ID"=w419) -> ("error out"=w427:errorcluster, "invalid Id"=w425:bool, "node ref"=w428:T2)  [unwired: 7 in]
        n163 = case shown="False" w425 {
          tunnel: [w436 w466] -> w429
          tunnel: w428 -> [w433 _]
          tunnel: w427 -> [w439 w466]
          tunnel: w424 -> [w440 _]
          tunnel: w423 -> [_ _]
          tunnel: w420 -> [w437 _]
          tunnel: w418 -> [w434 _]
          frame False {
            n164 = in-place {
              in-place-border: w440 -> [w464]
              in-place-border: w439 -> [w462]
              in-place-border: [w461] -> w435
              in-place-border: [w460] -> w438
              in-place-border: w437 -> [w459]
              in-place-border: w434 -> [w458]
              in-place-border: [w457] -> w432
              n165 = in-place-dvr #7(w433) -> (w465:refnum<class "NISE_CEF_Node.lvclass">)  [unwired: 1 out]
              n166 = call-dynamic "MenuHandler.vi"("tree control"=w458, "main message queue"=w464, "error in"=w462, "menu string"=w459, "NISE_CEF_Node in"=w465) -> ("error out"=w461:errorcluster, "refresh tree?"=w457:bool, "Unhandled"=w460:bool, "NISE_CEF_Node out"=w463:refnum<class "NISE_CEF_Node.lvclass">)  [unwired: 3 in]
              n167 = in-place-dvr #7(w463) -> (w431:T2)  [unwired: 1 out]
            }
            n168 = case shown="False" w438 {
              tunnel: w437 -> [_ w452]
              tunnel: [w444 w453] -> w436
              tunnel: w435 -> [w442 w454]
              tunnel: w432 -> [w441 _]
              tunnel: w431 -> [w443 _]
              frame False {
                n169 = case shown="True" w441 {
                  tunnel: [w445 w448] -> w444
                  tunnel: w443 -> [_ w447]
                  tunnel: w442 -> [w445 w446]
                  frame False {
                  }
                  frame True {
                    n170 = call <vilib>:"NodetoID.vi"("error in"=w446, "node ref"=w447) -> ("error out"=w450:errorcluster, "ID"=w451:string)  [unwired: 8 in]
                    n171 = call <vilib>:"Send Local Message.vi"("message name"="NodeDataChange", "message value"=w451, "error in"=w450) -> ("error out"=w448:errorcluster)  [unwired: 10 in, 2 out]
                  }
                }
              }
              frame True {
                n172 = call <vilib>:"NISE_error generator.vi"("error in"=w454, "source"="configuration tool main.vi", "append error message"=w452, "error code (0)"=538506) -> ("error out"=w453:errorcluster)  [unwired: 5 in]
              }
            }
          }
          frame True {
          }
        }
      }
      frame "RefreshNode" {
        # "Refreshes the node in the Tree, Sets the save flag to true. This case can be called from the UIs of the nodes"
        n173 = Unbundle By Name(w468) -> ("glyph manager"=w467:T9)
        n174 = call <vilib>:"IDtoNode.vi"("error in"=w475, "ID"=w473) -> ("error out"=w474:errorcluster, "invalid Id"=w471:bool, "node ref"=w472:T2)  [unwired: 7 in]
        n175 = case shown="False" w471 {
          tunnel: [w487 w490] -> w477
          tunnel: w474 -> [w483 w490]
          tunnel: w472 -> [w482 _]
          tunnel: w470 -> [w481 _]
          tunnel: [w480 w489] -> w469
          tunnel: w467 -> [w478 w489]
          frame False {
            n176 = call <vilib>:"SummaryWithGlyphManager.vi"("error in"=w483, "glyph manager"=w478, "node self ref"=w482) -> ("error out"=w485:errorcluster, "glyph manager out"=w479:T9, "summary"=w484:T18[])  [unwired: 6 in]
            n177 = call <vilib>:"RefreshSubTreeWithGlyphManager.vi"("error in"=w485, "glyph manager"=w479, "node information"=w484, "tree ref in"=w481) -> ("error out"=w488:errorcluster, "glyph manager out"=w480:T9, "tree ref out"=w486:refnum<vi>)  [unwired: 5 in]
            n178 = Close Reference(reference=w486, error in (no error)=w488) -> (error out=w487:errorcluster)
          }
          frame True {
          }
        }
        n179 = Bundle By Name(cluster=w468, "glyph manager"=w469) -> (w476:T1)
      }
      frame "RemoveNode" {
        n180 = call <vilib>:"IDtoNode.vi"("error in"=w496, "ID"=w497) -> ("error out"=w495:errorcluster, "invalid Id"=w492:bool, "node ref"=w494:T2)  [unwired: 7 in]
        n181 = case shown="False" w492 {
          tunnel: w495 -> [w504 w505]
          tunnel: w494 -> [w503 _]
          tunnel: [w500 w505] -> w493
          tunnel: w491 -> [w499 _]
          frame False {
            n182 = call <vilib>:"RemoveNode.vi"("error in"=w504, "node"=w503) -> ("error out"=w501:errorcluster, "node ID"=w502:string)  [unwired: 8 in]
            n183 = call <vilib>:"ClearTreeNode.vi"("error in"=w501, "tag"=w502, "tree reference"=w499) -> ("error out"=w500:errorcluster)  [unwired: 8 in]
          }
          frame True {
          }
        }
      }
      frame "PopulateTree" {
        n184 = Unbundle By Name(w521) -> ("standard events"=w511:T3, "glyph manager"=w507:T9, "root"=w516:T2)
        n185 = call <vilib>:"SummaryWithGlyphManager.vi"("error in"=w518, "glyph manager"=w507, "depth"=0 ("Depth"), "node self ref"=w516) -> ("error out"=w517:errorcluster, "glyph manager out"=w506:T9, "summary"=w520:T18[])  [unwired: 5 in]
        n186 = control-ref of="This VI"() -> (w519:refnum<vi>)
        n187 = call <vilib>:"RefreshEntireTreeWithGlyphManager.vi"("calling VI in"=w519, "error in"=w517, "glyph manager"=w506, "array"=w520, "tree ref in"=w510) -> ("error out"=w513:errorcluster, "glyph manager out"=w508:T9)  [unwired: 5 in]
        n188 = control-ref of="Sub Panel"() -> (w514:refnum<vi>)
        n189 = call <vilib>:"ClearSubPanelStandardEvents.vi"("error in"=w513, "standard events"=w511, "sub panel ref in"=w514) -> ("error out"=w512:errorcluster)  [unwired: 7 in, 1 out]
        n190 = Bundle By Name(cluster=w521, "glyph manager"=w508) -> (w509:T1)
      }
      frame "CleansubPanel" {
        n191 = Unbundle By Name(w526) -> ("standard events"=w522:T3)
        n192 = control-ref of="Sub Panel"() -> (w528:refnum<vi>)
        n193 = call <vilib>:"ClearSubPanelStandardEvents.vi"("error in"=w527, "standard events"=w522, "sub panel ref in"=w528) -> ("error out"=w525:errorcluster, "sub panel ref out"=w524:refnum<vi>)  [unwired: 7 in]
        n194 = Close Reference(reference=w524, error in (no error)=w525) -> (error out=w523:errorcluster)
      }
      frame "ActivateNode" {
        n195 = Unbundle By Name(w531) -> ("standard events"=w530:T3)
        n196 = call <vilib>:"IDtoNode.vi"("error in"=w536, "ID"=w537) -> ("error out"=w529:errorcluster, "invalid Id"=w535:bool, "node ref"=w534:T2)  [unwired: 7 in]
        n197 = case shown="False" w535 {
          tunnel: w534 -> [w544 _]
          tunnel: [w545 w546] -> w533
          tunnel: w529 -> [w542 w546]
          tunnel: w532 -> [w540 _]
          tunnel: w530 -> [w538 _]
          frame False {
            n198 = control-ref of="Sub Panel"() -> (w541:refnum<vi>)
            n199 = call <vilib>:"ClearSubPanelStandardEvents.vi"("error in"=w542, "standard events"=w538, "sub panel ref in"=w541) -> ("error out"=w543:errorcluster, "sub panel ref out"=w539:refnum<vi>)  [unwired: 7 in]
            n200 = call <vilib>:"LoadNodeUIStandardEvents.vi"("user event out"=w538, "error in"=w543, "sub panel ref in"=w539, "main queue"=w540, "node"=w544) -> ("error out"=w545:errorcluster)  [unwired: 6 in]
          }
          frame True {
          }
        }
      }
      frame "Move" {
        n201 = Unflatten From String(type=T14 {"node ref"=refnum, "new parent"=refnum, "Index"=0} ("Cluster"), binary string=w558, error in (no error)=w556) -> (value=w555:T14, error out=w554:errorcluster)  [unwired: 2 in, 1 out]
        n202 = Unbundle By Name(w555) -> ("node ref"=w549:T2, "new parent"=w548:T2, "Index"=w547:i32)
        n203 = call <vilib>:"MoveNode.vi"("error in"=w554, "index"=w547, "new parent"=w548, "node"=w549) -> ("error out"=w552:errorcluster)  [unwired: 7 in]
        n204 = call <vilib>:"Send Local Message.vi"("message queue in"=w550, "message name"="PopulateTree", "error in"=w552) -> ("error out"=w551:errorcluster)  [unwired: 10 in, 2 out]
      }
      frame "NodeDataChange" {
        n205 = call <vilib>:"Send Local Message.vi"("message queue in"=w563, "message name"="RefreshNode", "message value"=w565, "error in"=w566) -> ("error out"=w564:errorcluster)  [unwired: 9 in, 2 out]
        n206 = Bundle By Name(cluster=w567, "unsaved changes"=TRUE) -> (w561:T1)
      }
    }
  }
  n207 = while "User Interface Event Handler" {
    tunnel: w14 -> [w574]
    tunnel: w13 -> [w570]
    tunnel: w5 -> [w569]
    tunnel: [w568] -> w1
    stop <- w573 stop-if-true
    n208 = event shown="[6] \"View\": Value Change" {
      selector: w569 -> [_ _ _ _ _ _ _ _ _ _ _]
      dyn-events: [_ _ _ _ _ _ _ _ _ _ _] -> w568
      timeout: 250 -> [_ _ _ _ _ _ _ _ _ _ _]
      tunnel: w574 -> [w577 w585 w609 w659 w688 w695 w724 w729 w739 w745 w791]
      tunnel: [_ _ _ _ TRUE _ _ _ _ _ _] -> w573
      tunnel: [w577 w585 w606 w657 w684 w695 w721 w729 w737 w744 w792] -> w572
      tunnel: [w576 w581 w605 w656 w685 w691 w720 w726 w735 w742 _] -> w571
      tunnel: w570 -> [w576 w584 w604 w658 w686 w694 w719 w728 w736 w743 _]
      event Timeout {
        # "Timeout code can be added here for autosave or Lock Screen"
        n209 = event-data() -> ()  [unwired: 1 in, 1 out]
      }
      event "View": Shortcut Menu Activation? {
        n210 = event-data() -> ("CtlRef"=w591:refnum<vi>, "Coords"=w590:T19, "MenuRef"=w587:refnum<k9>)  [unwired: 1 in]
        n211 = invoke class="Tree (strict)" method="Point To Row Column"(reference=w591, error in=w584, "Point"=w590) -> (error out=w583:errorcluster, "Tag"=w589:string)  [unwired: 5 in, 6 out]
        n212 = call <vilib>:"IDtoNode.vi"("error in"=w583, "ID"=w589) -> ("error out"=w579:errorcluster, "invalid Id"=w586:bool, "node ref"=w588:T2)  [unwired: 7 in]
        n213 = case shown="False" w586 {
          tunnel: w588 -> [w596 _]
          tunnel: w587 -> [w595 _]
          tunnel: [w594 _] -> w582
          tunnel: [w593 _] -> w580
          tunnel: w579 -> [w592 w602]
          tunnel: [w592 w602] -> w578
          frame False {
            n214 = in-place {
              in-place-border: w595 -> [w599]
              in-place-border: [w597] -> w594
              n215 = in-place-dvr #8(w596) -> (w601:refnum<class "NISE_CEF_Node.lvclass">, w598:errorcluster)
              n216 = call-dynamic "ShortcutMenu.vi"("error in"=w598, "menu ref in"=w599, "node in"=w601) -> ("error out"=w597:errorcluster, "node out"=w600:refnum<class "NISE_CEF_Node.lvclass">)  [unwired: 6 in, 1 out]
              n217 = in-place-dvr #8(w600) -> (w593:errorcluster)  [unwired: 1 out]
            }
          }
          frame True {
          }
        }
        n218 = Merge Errors(w580, w582, w578) -> (w581:errorcluster)
        n219 = event-data() -> ()  [unwired: 2 in, 1 out]
      }
      event "View": Shortcut Menu Selection (User) {
        n220 = event-data() -> ("ItemPath"=w608:string, "CtlRef"=w612:refnum<vi>, "Coords"=w613:T19)  [unwired: 1 in]
        n221 = invoke class="Tree (strict)" method="Point To Row Column"(reference=w612, error in=w604, "Point"=w613) -> (error out=w603:errorcluster, "Tag"=w607:string)  [unwired: 5 in, 6 out]
        n222 = Match Pattern(string=w608, regular expression=":") -> (before substring=w611:string, after substring=w610:string)  [unwired: 1 in, 2 out]
        n223 = case shown="\"Add\", \"AddPeer\"" w611 {
          selector: w611 -> [w615 _ _ w636]
          tunnel: w610 -> [_ _ _ w637]
          tunnel: w609 -> [w622 w629 w635 w642]
          tunnel: w607 -> [w617 w627 w633 w641]
          tunnel: [w619 w626 w632 w640] -> w606
          tunnel: [w620 w625 w630 w638] -> w605
          tunnel: w603 -> [w621 w624 w631 w639]
          frame Default {
            n224 = Concatenate Strings(w615, ":" ("string"), w617) -> (w618:string)
            n225 = call <vilib>:"Send Local Message.vi"("message queue in"=w622, "message name"="CustomMenuAction" ("Message Name"), "message value"=w618, "error in"=w621) -> ("message queue out"=w619:T12, "error out"=w620:errorcluster)  [unwired: 9 in, 1 out]
          }
          frame "Remove" {
            n226 = call <vilib>:"Send Local Message.vi"("message queue in"=w629, "message name"="RemoveNode" ("Message Name"), "message value"=w627, "error in"=w624) -> ("message queue out"=w626:T12, "error out"=w625:errorcluster)  [unwired: 9 in, 1 out]
          }
          frame "Duplicate" {
            n227 = call <vilib>:"Send Local Message.vi"("message queue in"=w635, "message name"="Duplicate" ("Message Name"), "message value"=w633, "error in"=w631) -> ("message queue out"=w632:T12, "error out"=w630:errorcluster)  [unwired: 9 in, 1 out]
          }
          frame "Add", "AddPeer" {
            n228 = Bundle By Name(cluster=T13 {"node type"="", "to add to"=""} ("input cluster"), "node type"=w637, "to add to"=w641) -> (w643:T13)
            n229 = Flatten To String(anything=w643) -> (data string=w644:string)  [unwired: 3 in, 2 out]
            n230 = call <vilib>:"Send Local Message.vi"("message queue in"=w642, "message name"=w636, "message value"=w644, "error in"=w639) -> ("message queue out"=w640:T12, "error out"=w638:errorcluster)  [unwired: 9 in, 1 out]
          }
        }
      }
      event "View": Drop {
        n231 = event-data() -> ("CtlRef"=w662:refnum<vi>, "Coords"=w661:T19)  [unwired: 1 in]
        n232 = invoke class="Tree (strict)" method="Point To Row Column"(reference=w662, error in=w658, "Point"=w661) -> (reference out=w660:refnum<vi>, error out=w655:errorcluster, "Tag"=w652:string)  [unwired: 5 in, 5 out]
        n233 = call <vilib>:"ValidDragDrop.vi"("error in"=w655, "Reorder"=TRUE, "drag over"=w652, "Tree Ref in"=w660) -> ("Error Out"=w647:errorcluster, "Accepted"=w650:bool, "Drag"=w654:string, "Tree Ref out"=w664:refnum<vi>, "Moved Node"=w648:T2, "Position"=w646:i32, "Parent Node"=w649:T2, "Parent"=w651:string)
        n234 = case shown="True" w650 {
          tunnel: w654 -> [_ w681]
          tunnel: w664 -> [_ w683]
          tunnel: [_ TRUE] -> w663
          tunnel: w651 -> [_ w679]
          tunnel: w659 -> [w666 w678]
          tunnel: [w666 w674] -> w657
          tunnel: [w665 w673] -> w656
          tunnel: w648 -> [_ w669]
          tunnel: w649 -> [_ w668]
          tunnel: w647 -> [w665 w670]
          tunnel: w646 -> [_ w667]
          frame False {
          }
          frame True {
            n235 = invoke class="Tree (strict)" method="Edit Tree Items.Move Item"(reference=w683, error in=w670, "tag"=w681, "New Parent"=w679) -> (error out=w671:errorcluster)  [unwired: 3 in, 6 out]
            n236 = Bundle By Name(cluster=T14 {"node ref"=refnum, "new parent"=refnum, "Index"=0} ("Cluster"), "Index"=w667, "node ref"=w669, "new parent"=w668) -> (w677:T14)
            n237 = Flatten To String(anything=w677, error in (no error)=w671) -> (data string=w676:string, error out=w672:errorcluster)  [unwired: 2 in, 1 out]
            n238 = call <vilib>:"Send Local Message.vi"("message queue in"=w678, "message name"="Move", "message value"=w676, "error in"=w672) -> ("message queue out"=w674:T12, "error out"=w673:errorcluster)  [unwired: 9 in, 1 out]
          }
        }
        n239 = event-data("Accepted?"=w663) -> ()  [unwired: 1 in, 1 out]
      }
      event "Exit": Value Change {
        # "Exit the application                                           >> Stop this message generator loop    Cleaning errors if the other loop stop this one"
        n240 = event-data() -> ()  [unwired: 1 in, 1 out]
        n241 = call <vilib>:"Send Local Message.vi"("message queue in"=w688, "message name"="Close", "error in"=w686) -> ("message queue out"=w684:T12, "error out"=w689:errorcluster)  [unwired: 10 in, 1 out]
        n242 = call <vilib>:"Clear Errors.vi"("error in (no error)"=w689) -> ("error out"=w685:errorcluster)  [unwired: 5 in, 1 out]
      }
      event "View": Drag Starting? {
        n243 = event-data() -> ("Data"=w701:T20, "CtlRef"=w703:refnum<vi>, "Coords"=w702:T19)  [unwired: 1 in]
        n244 = invoke class="Tree (strict)" method="Point To Row Column"(reference=w703, error in=w694, "Point"=w702) -> (error out=w693:errorcluster, "Tag"=w700:string)  [unwired: 5 in, 6 out]
        n245 = call <vilib>:"IDtoNode.vi"("error in"=w693, "ID"=w700) -> ("error out"=w692:errorcluster, "invalid Id"=w699:bool, "node ref"=w698:T2)  [unwired: 7 in]
        n246 = case shown="True" w699 {
          tunnel: w698 -> [w711 _]
          tunnel: [w708 TRUE ("Removable")] -> w696
          tunnel: w692 -> [w707 w717]
          tunnel: [w704 w717] -> w691
          frame False {
            n247 = in-place {
              in-place-border: [w714] -> w710
              in-place-border: w707 -> [w713]
              in-place-border: [w712] -> w706
              n248 = in-place-dvr #9(w711) -> (w716:refnum<class "NISE_CEF_Node.lvclass">)  [unwired: 1 out]
              n249 = call-dynamic "EditOptions.vi"("error in"=w713, "node in"=w716) -> ("error out"=w712:errorcluster, "edit options"=w714:T21, "node out"=w715:refnum<class "NISE_CEF_Node.lvclass">)  [unwired: 6 in, 1 out]
              n250 = in-place-dvr #9(w715) -> (w705:errorcluster)  [unwired: 1 out]
            }
            n251 = Unbundle By Name(w710) -> ("movable"=w709:bool)
            n252 = Merge Errors(w705, w706) -> (w704:errorcluster)
            n253 = Not(x=w709) -> (.not. x?=w708:bool)
          }
          frame True {
          }
        }
        n254 = event-data("Data"=w701, "Drag Mode"=enum32{"copy or move", "copy only", "move only"}."move only", "Discard?"=w696) -> ()  [unwired: 1 in, 1 out]
      }
      event "View": Value Change {
        n255 = event-data() -> ("NewVal"=w722:string)  [unwired: 1 in]
        n256 = call <vilib>:"Send Local Message.vi"("message queue in"=w724, "message name"="ActivateNode" ("Message Name"), "message value"=w722, "error in"=w719) -> ("message queue out"=w721:T12, "error out"=w720:errorcluster)  [unwired: 9 in, 1 out]
      }
      event "View": event type 3.0.xa000003a {
        n257 = event-data() -> ("CtlRef"=w734:refnum<vi>, "Coords"=w731:T19)  [unwired: 1 in]
        n258 = invoke class="Tree (strict)" method="Point To Row Column"(reference=w734, error in=w728, "Point"=w731) -> (reference out=w733:refnum<vi>, error out=w727:errorcluster, "Tag"=w732:string)  [unwired: 5 in, 5 out]
        n259 = call <vilib>:"ValidDragDrop.vi"("error in"=w727, "Reorder"=TRUE, "drag over"=w732, "Tree Ref in"=w733) -> ("Error Out"=w726:errorcluster, "Accepted"=w730:bool)  [unwired: 6 out]
        n260 = event-data("Accepted?"=w730) -> ()  [unwired: 1 in, 1 out]
      }
      event Panel Close? {
        # "Intercepts the upper right close panel operation to allow a smooth shutdown as opposed to immediately killing the app."
        n261 = event-data() -> ()  [unwired: 1 in, 1 out]
        n262 = call <vilib>:"Send Local Message.vi"("message queue in"=w739, "message name"="Close?", "error in"=w736) -> ("message queue out"=w737:T12, "error out"=w735:errorcluster)  [unwired: 10 in, 1 out]
        n263 = event-data("Discard?"=TRUE) -> ()  [unwired: 1 in, 1 out]
      }
      event Menu Selection (User) {
        # "#USERCFG It is needed to add a Case for Every item on the menu"
        n264 = event-data() -> ("ItemTag"=w741:string, "ItemPath"=w746:string)  [unwired: 1 in]
        n265 = case shown="\"_File:_Save\"" w746 {
          selector: w746 -> [w750 _ _ _ _ _ _]
          tunnel: w745 -> [w755 w760 w765 w770 w775 w780 w789]
          tunnel: [w755 w756 w761 w766 w771 w776 w786] -> w744
          tunnel: w743 -> [w752 w758 w763 w768 w773 w778 w785]
          tunnel: [w751 w757 w762 w767 w772 w777 w783] -> w742
          tunnel: w741 -> [w749 _ _ _ _ _ _]
          frame Default {
            n266 = Concatenate Strings(w749, "::" ("string"), w750) -> (w748:string)
            n267 = call <vilib>:"NISE_error generator.vi"("error in"=w752, "source"="configuration tool main.vi", "append error message"=w748, "error code (0)"=538506) -> ("error out"=w751:errorcluster)  [unwired: 5 in]
          }
          frame "_File:_New" {
            n268 = call <vilib>:"Send Local Message.vi"("message queue in"=w760, "message name"="New?" ("Message Name"), "error in"=w758) -> ("message queue out"=w756:T12, "error out"=w757:errorcluster)  [unwired: 10 in, 1 out]
          }
          frame "_File:_Open" {
            n269 = call <vilib>:"Send Local Message.vi"("message queue in"=w765, "message name"="Open?" ("Message Name"), "error in"=w763) -> ("message queue out"=w761:T12, "error out"=w762:errorcluster)  [unwired: 10 in, 1 out]
          }
          frame "_File:_Save" {
            n270 = call <vilib>:"Send Local Message.vi"("message queue in"=w770, "message name"="Save" ("Message Name"), "error in"=w768) -> ("message queue out"=w766:T12, "error out"=w767:errorcluster)  [unwired: 10 in, 1 out]
          }
          frame "_File:Save As..." {
            n271 = call <vilib>:"Send Local Message.vi"("message queue in"=w775, "message name"="SaveAs" ("Message Name"), "error in"=w773) -> ("message queue out"=w771:T12, "error out"=w772:errorcluster)  [unwired: 10 in, 1 out]
          }
          frame "_File:_Exit" {
            n272 = call <vilib>:"Send Local Message.vi"("message queue in"=w780, "message name"="Close?" ("Message Name"), "error in"=w778) -> ("message queue out"=w776:T12, "error out"=w777:errorcluster)  [unwired: 10 in, 1 out]
          }
          frame "_Tools:Multiple Parameter Editor" {
            n273 = call <vilib>:"Send Local Message.vi"("message queue in"=w789, "message name"="CleansubPanel", "error in"=w785) -> ("message queue out"=w788:T12, "error out"=w784:errorcluster)  [unwired: 10 in, 1 out]
            n274 = call <vilib>:"Send Local Message.vi"("message queue in"=w788, "message name"="Custom View" ("Message Name"), "message value"="Multiple Variable Editor" ("Message Name"), "error in"=w784) -> ("message queue out"=w786:T12, "error out"=w783:errorcluster)  [unwired: 9 in, 1 out]
          }
        }
      }
      event User Event {
        n275 = event-data() -> ("node ref"=w790:T2)  [unwired: 1 in]
        n276 = call <vilib>:"NodetoID.vi"("node ref"=w790) -> ("ID"=w793:string)  [unwired: 9 in, 1 out]
        n277 = call <vilib>:"Send Local Message.vi"("message queue in"=w791, "message name"="NodeDataChange", "message value"=w793) -> ("message queue out"=w792:T12)  [unwired: 10 in, 2 out]
      }
    }
    n278 = call "Error.vi"("error in (no error)"=w571, "message queue in"=w572) -> ()  [unwired: 9 in, 1 out]
  }
  n279 = Unregister For Events(event registration refnum=w1) -> (error out=w2:errorcluster)  [unwired: 1 in]
  n280 = Merge Errors(w2, w7) -> (w3:errorcluster)
  n281 = call <vilib>:"DestroyStandardEvents.vi"("error in"=w3, "standard events"=w6) -> ()  [unwired: 9 in, 1 out]
